vi "123.vi"() -> ()   [LabVIEW 2014]
panel:
  in  "Path to Save Report":path=path "C:/Users/Administrator/Desktop/报表/123.doc"
  out "Saved Report Path":path
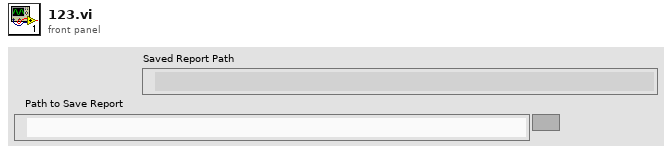
[diagram p1: front panel]
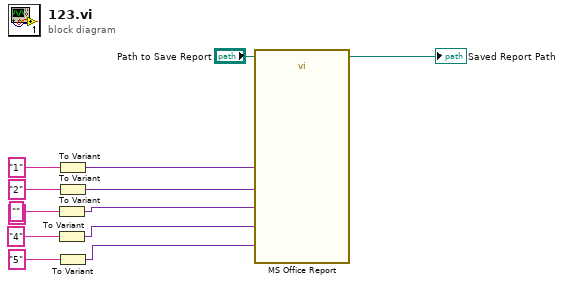
[diagram p0: block diagram]
diagram:
  (unwired) "3"
  n1 = To Variant(anything="") -> (Variant=w7:variant)
  n2 = To Variant(anything="4") -> (Variant=w5:variant)
  n3 = To Variant(anything="1") -> (Variant=w11:variant)
  n4 = To Variant(anything="2") -> (Variant=w9:variant)
  n5 = To Variant(anything="5") -> (Variant=w3:variant)
  n6 = call "MS Office Report"("Path to Save Report"="Path to Save Report", "名称"=w11, "型号"=w9, "尺寸"=w7, "日期"=w5, "长度"=w3) -> ("Saved Report Path"=→"Saved Report Path":path)  [unwired: 20 in, 1 out]
